vi "Output_RC.vi"(0 "Rack Controller in":refnum<class "Rack Controller.lvclass">, 5 "Output Cluster":T1={"Acknowledgement"={"Actor Enqueuer"=refnum, "VI Reference"=refnum, "VI Name"=""}, "Rack ID"=0, "Clear"=FALSE, "Light Camera Info"={"Light Camera Name"="", " State"=""}, "Camera Optics Diagnostics Result"={"LightCameraName"="", "DiagnosedImage"=refnum, "DustPercentage"=0.0, "Result"=TRUE}, "Receiver Enqueuer"={"Actor Enqueuer"=refnum, "VI Name"=""}, "Error Message"="", "Part Details"={"Part Name"="", "Total Count"=0, "Reel Count"=0}, "Result Cluster"={"RackID"=0, "MeasurementValuesArray "=[], "ImagesArray"=[], "ResultPF"=FALSE, "ProductionCountDetails"={"TotalFail"=0, "TotalPass"=0, "TotalCount"=0}, "ReelCountDetails"={"ReelFail"=0, "ReelPass"=0, "ReelCount"=0}, "ControlPFArray"=[], "SpecificationPFArray"=[], "SpecificationFail"=FALSE, "ReelNumber"=0, "Status"=""}, "Part Info"={"Part Name"="", "Rack ID"=0, "MeasurementIDsArray"=[], "Measurement Names Array"=[], "Spec Values Array"=[], "Camera Names Array"=[], "Total count"=0, "Reel count"=0}, "AllPartInfo"=[{"PartName"="", "NumberOfRacks"=0, "MeasurementIDsArray"=[], "MeasurementNamesArray"=[], "SpecValuesArray"=[]}], "ImagesAndCount"={"Image Array"=[], "ImageCount"=0}}, 7 "Receiver Name":string(combo), 9 "State":string, 11 "error in (no error)":errorcluster) -> (15 "error out":errorcluster)   [LabVIEW 2019, in "Rack Controller.lvclass"]
uses:
  Rack Controller.lvclass
  Inspection Statemachine/Inspection Statemachine Messages/Acknowledgement_SM Msg/Acknowledgement_SM.lvclass
  <vilib>/ActorFramework/Actor/Actor.lvclass
  Inspection Statemachine/Inspection Statemachine Messages/Clear_SM Msg/Clear_SM Msg.lvclass
  Inspection Statemachine/Inspection Statemachine Messages/ErrorMessage_SM Msg/ErrorMessage_SM Msg.lvclass
  Inspection Statemachine/Inspection Statemachine Messages/ResultData_SM Msg/ResultData_SM Msg.lvclass
  <vilib>/ActorFramework/Message Enqueuer/Message Priority.ctl
  <vilib>/ActorFramework/Message Enqueuer/Message Enqueuer.lvclass
  Algorithm/Algorithm Messages/PartInfo_Algo Msg/PartInfo_Algo Msg.lvclass
  Algorithm/Algorithm Messages/StateMessage_Algo Msg/StateMessage_Algo Msg.lvclass
  Algorithm/Algorithm Messages/RackID_Algo Msg/RackID_Algo Msg.lvclass
  Inspection Statemachine/Inspection Statemachine Messages/AllPartInfo_SM Msg/AllPartInfo_SM Msg.lvclass
  Inspection Statemachine/Inspection Statemachine Messages/SensorDiagnosticsResult_SM Msg/SensorDiagnosticsResult_SM Msg.lvclass
  ZenCAM/Camera Controller/Camera Controller Messages/State Message CC Msg/State Message CC Msg.lvclass
  ZenCAM/Camera Controller/Camera Controller Messages/Camera Contoller ID CC Msg/Camera Contoller ID CC Msg.lvclass
  ZenCAM/Camera Controller/Camera Controller Messages/Camera Optics Diagnostics Msg/Camera Optics Diagnostics CC Msg.lvclass
  Inspection Statemachine/Inspection Statemachine Messages/CameraOpticsDiagnosticsResult_SM Msg/CameraOpticsDiagnosticsResult_SM Msg.lvclass
  ZenCAM/Camera Controller/Camera Controller Messages/Reciever Enqueuer CC Msg/Reciever Info CC Msg.lvclass
  ZenCAM/Camera Controller/Camera Controller Messages/Part Name CC Msg/Part Name CC Msg.lvclass
  ZenCAM/Camera Controller/Camera Controller Messages/Run CC Msg/Run CC Msg.lvclass
  Inspection Statemachine/Inspection Statemachine Messages/PartInfoInit_SM Msg/PartInfo_SM Msg.lvclass
  C:/Program Files/National Instruments/LabVIEW 2019/vi.lib/ActorFramework/Actor/Actor.lvclass
  Controls/Output Cluster_RC.ctl
  <vilib>/vision/Image Controls.llb/IMAQ Image.ctl
  Common/Controls/Camera Optics Diagnostics.ctl
  Common/Controls/Camera Optics Diagnostics Result.ctl
  Inspection Statemachine/Controls/Result Cluster_SM.ctl
  Inspection Statemachine/Inspection Statemachine.lvclass
  Common/Controls/AllPartInfo.ctl
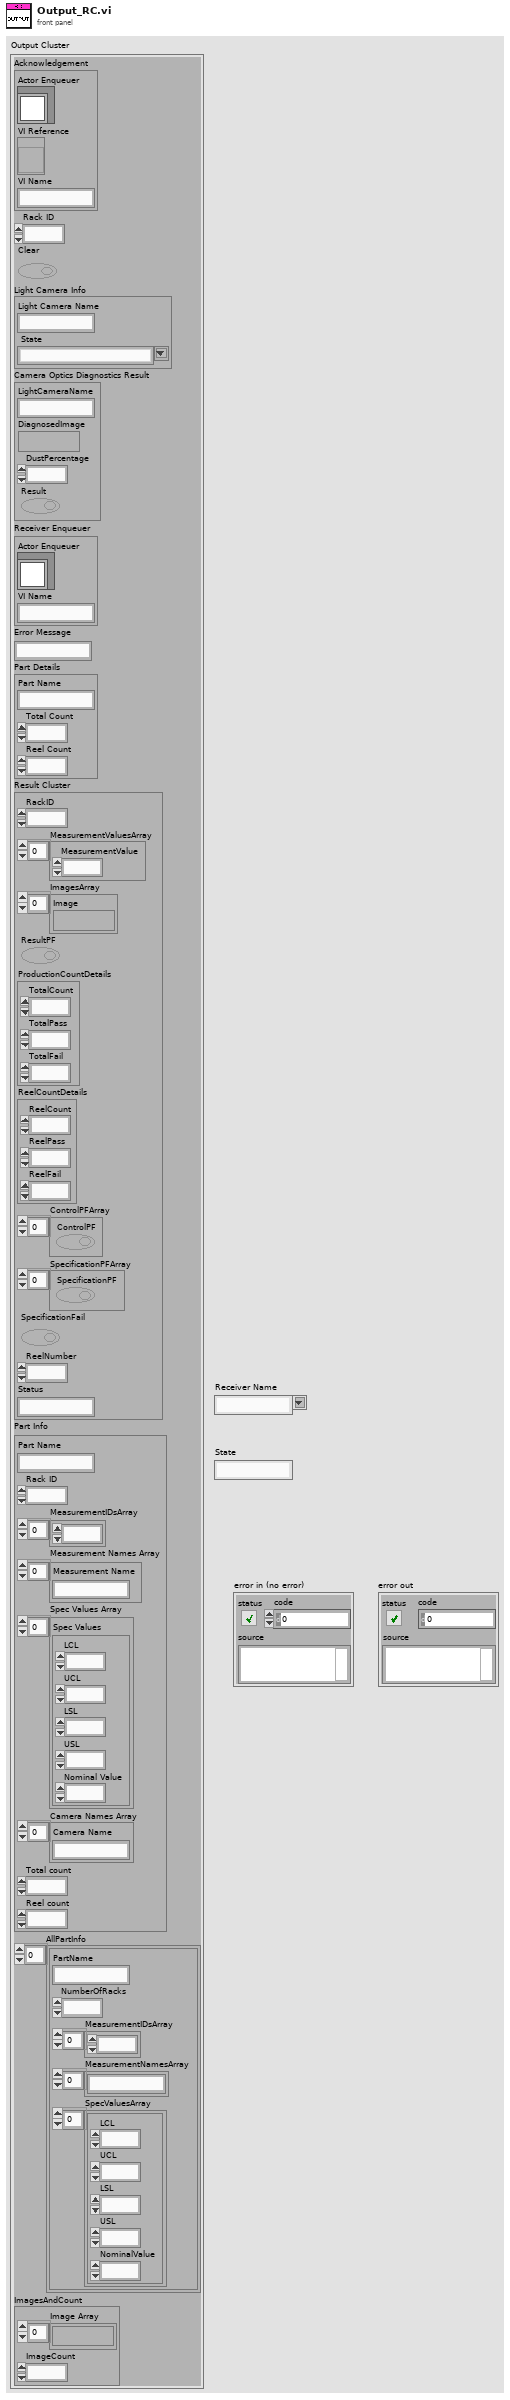
[diagram p1: front panel]
types:
  T1 = typedef "Rack Controller.lvclass/Output Cluster_RC.ctl" = cluster{"Acknowledgement":cluster{"Actor Enqueuer":refnum<class "Message Enqueuer.lvclass">, "VI Reference":refnum<vi>, "VI Name":string}, "Rack ID":u8, "Clear":bool, "Light Camera Info":T2, "Camera Optics Diagnostics Result":T3, "Receiver Enqueuer":cluster{"Actor Enqueuer":refnum<class "Message Enqueuer.lvclass">, "VI Name":string}, "Error Message":string, "Part Details":cluster{"Part Name":string, "Total Count":u64, "Reel Count":u64}, "Result Cluster":T5, "Part Info":cluster{"Part Name":string, "Rack ID":u8, "MeasurementIDsArray":u16[], "Measurement Names Array":string[], "Spec Values Array":cluster{"LCL":dbl, "UCL":dbl, "LSL":dbl, "USL":dbl, "Nominal Value":dbl}[], "Camera Names Array":string[], "Total count":u64, "Reel count":u64}, "AllPartInfo":T6, "ImagesAndCount":cluster{"Image Array":T4[], "ImageCount":u64}}
  T2 = typedef "Camera Optics Diagnostics.ctl" = cluster{"Light Camera Name":string, " State":string}
  T3 = typedef "Camera Optics Diagnostics Result.ctl" = cluster{"LightCameraName":string, "DiagnosedImage":T4, "DustPercentage":dbl, "Result":bool}
  T4 = typedef "IMAQ Image.ctl" = refnum<image>
  T5 = typedef "Inspection Statemachine.lvclass/Result Cluster_SM.ctl" = cluster{"RackID":u8, "MeasurementValuesArray ":dbl[], "ImagesArray":T4[], "ResultPF":bool, "ProductionCountDetails":cluster{"TotalFail":u64, "TotalPass":u64, "TotalCount":u64}, "ReelCountDetails":cluster{"ReelFail":u64, "ReelPass":u64, "ReelCount":u64}, "ControlPFArray":bool[], "SpecificationPFArray":bool[], "SpecificationFail":bool, "ReelNumber":u64, "Status":string}
  T6 = typedef "AllPartInfo.ctl" = cluster{"PartName":string, "NumberOfRacks":u8, "MeasurementIDsArray":u16[], "MeasurementNamesArray":string[], "SpecValuesArray":cluster{"LCL":dbl, "UCL":dbl, "LSL":dbl, "USL":dbl, "NominalValue":dbl}[]}[]
  T7 = typedef "Actor Framework.lvlib/Message Enqueuer.lvclass/Message Priority.ctl" = enum16{"Low", "Normal", "High"}
  T8 = cluster{"State":string, "Image File path":cluster{"Path":path, "Camera ID":i32}[]}
  T9 = cluster{"Reciever Enqueuers":refnum<class "Message Enqueuer.lvclass">, "Recievers Name":string, "Recievers ID":i32}
  T10 = cluster{"Totalcount":u64, "Reelcount":u64, "PartName":string}
  T11 = cluster{"PartName":string, "RackID":u8, "Re-Initialize":bool, "MeasurementIDsArray":u16[], "MeasurementNamesArray":string[], "SpecValuesArray":cluster{"LCL":dbl, "UCL":dbl, "LSL":dbl, "USL":dbl, "NominalValue":dbl}[], "CameraNamesArray":string[]}
  T12 = cluster{"Actor Enqueuer":refnum<class "Message Enqueuer.lvclass">, "VI Reference":refnum<vi>, "VI Name":string}
  T13 = cluster{"LCL":dbl, "UCL":dbl, "LSL":dbl, "USL":dbl, "Nominal Value":dbl}[]
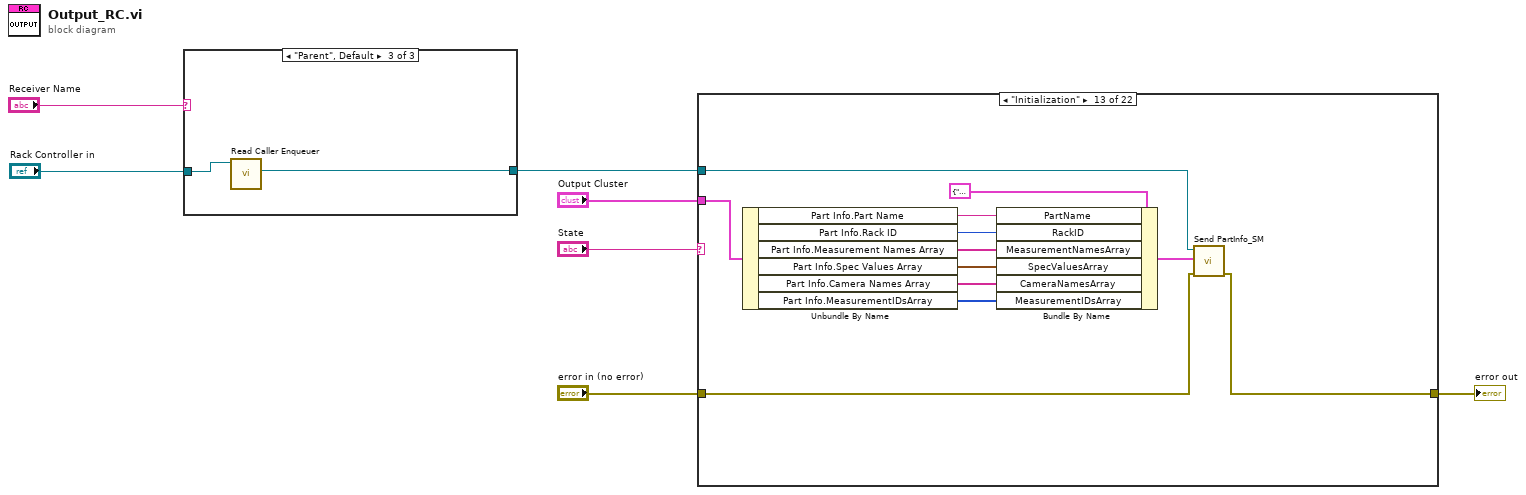
[diagram p0: block diagram]
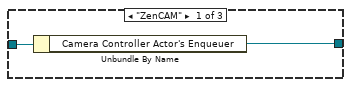
[diagram p2: hidden frame]
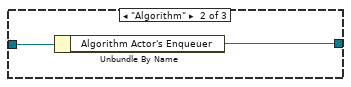
[diagram p3: hidden frame]
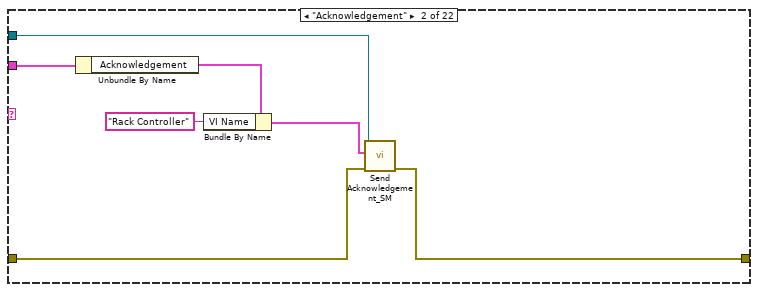
[diagram p5: hidden frame]
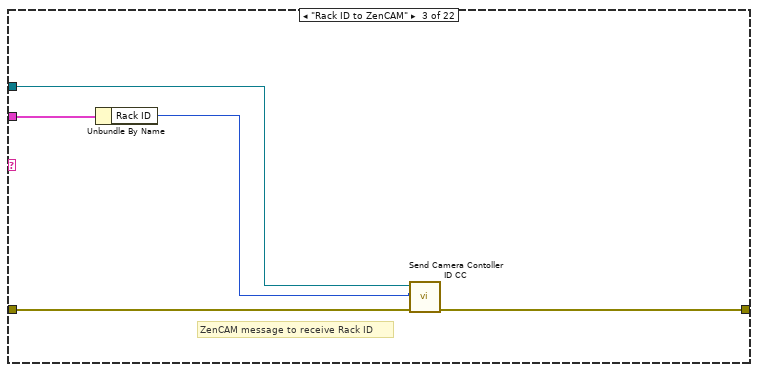
[diagram p6: hidden frame]
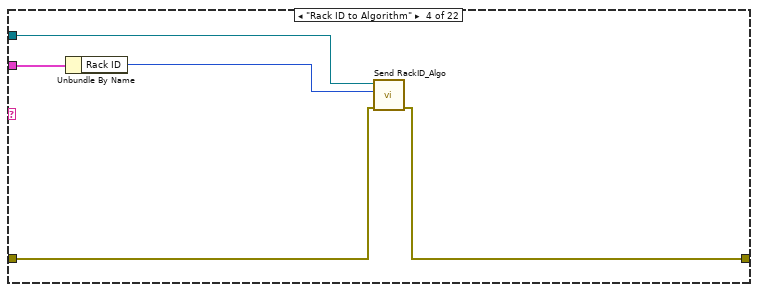
[diagram p7: hidden frame]
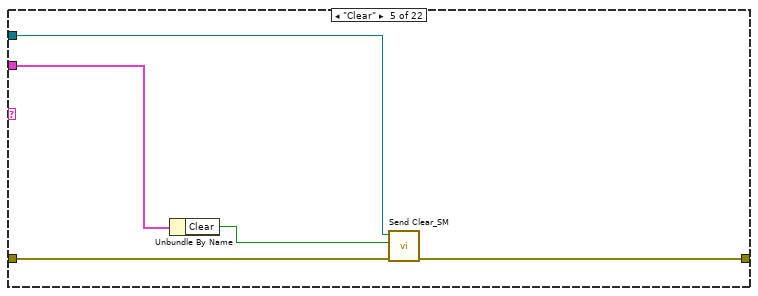
[diagram p8: hidden frame]
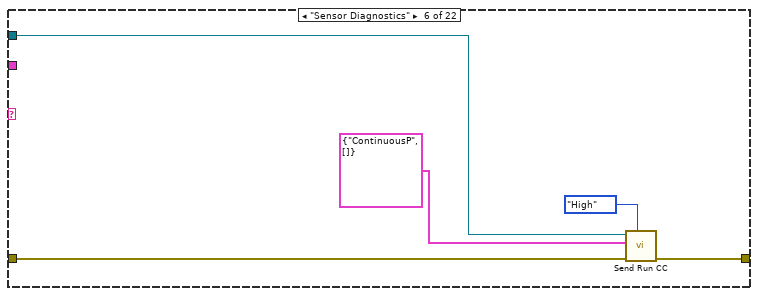
[diagram p9: hidden frame]
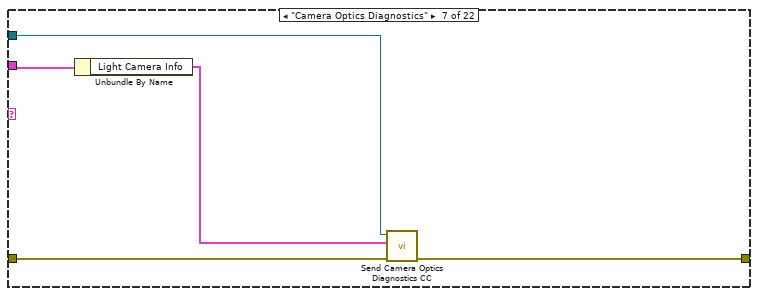
[diagram p10: hidden frame]
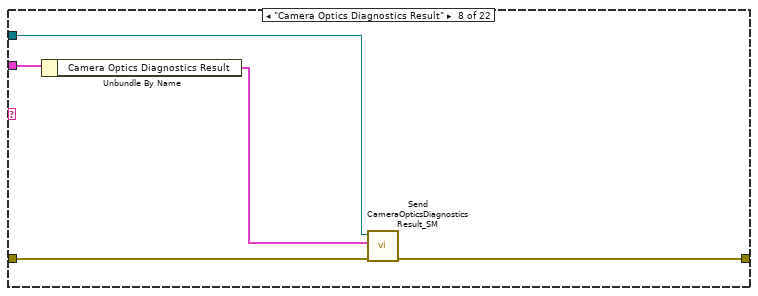
[diagram p11: hidden frame]
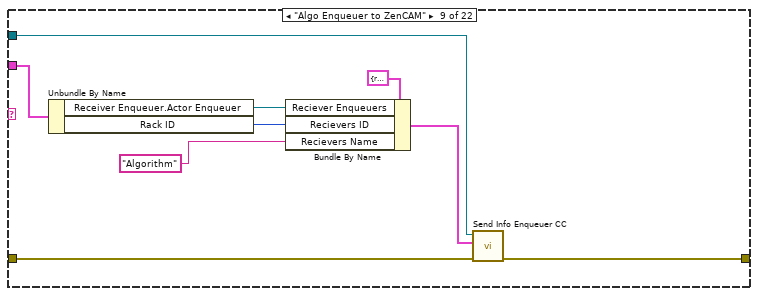
[diagram p12: hidden frame]
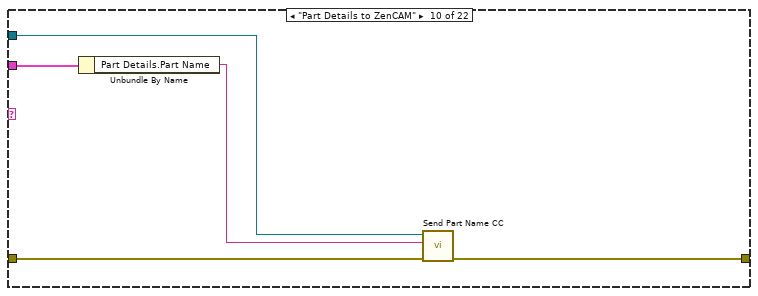
[diagram p13: hidden frame]
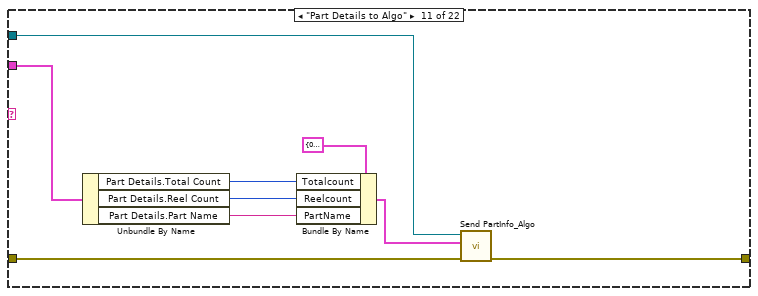
[diagram p14: hidden frame]
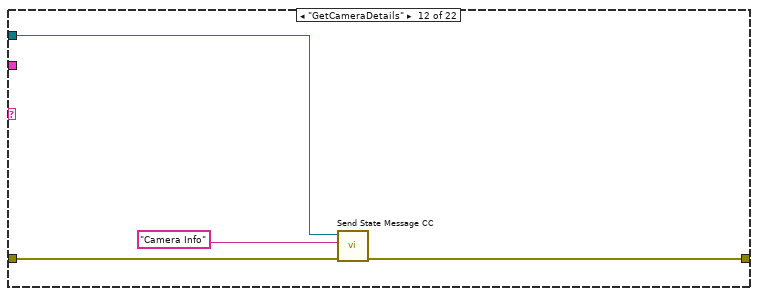
[diagram p15: hidden frame]
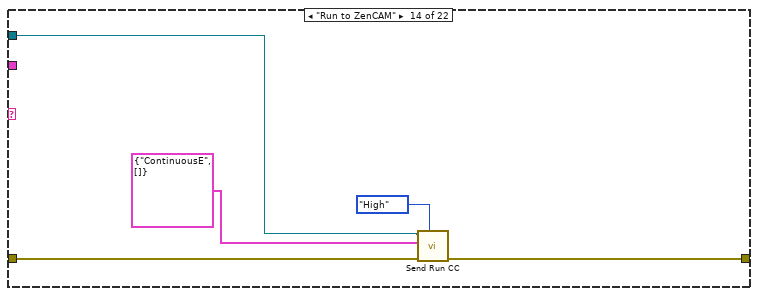
[diagram p16: hidden frame]
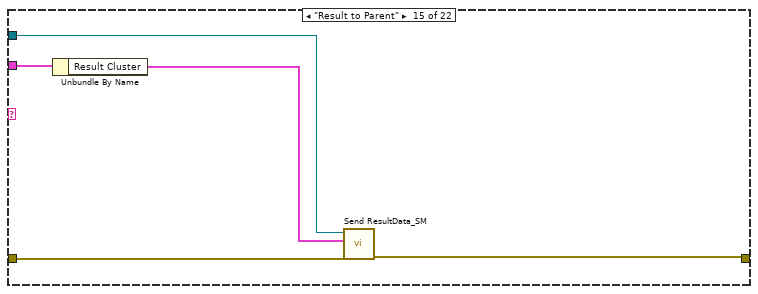
[diagram p17: hidden frame]
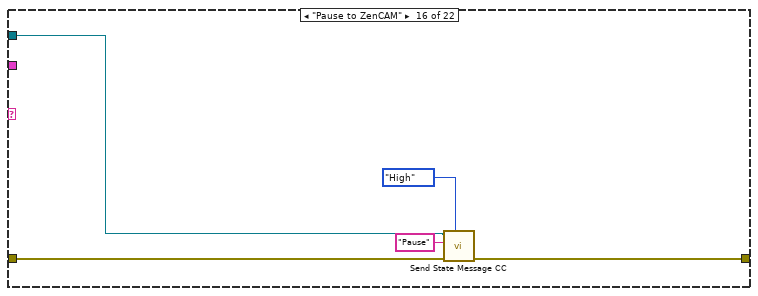
[diagram p18: hidden frame]
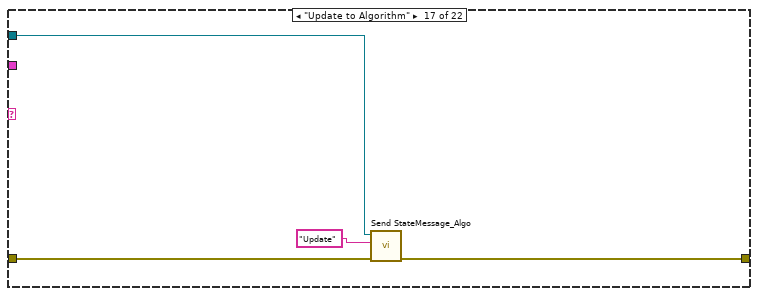
[diagram p19: hidden frame]
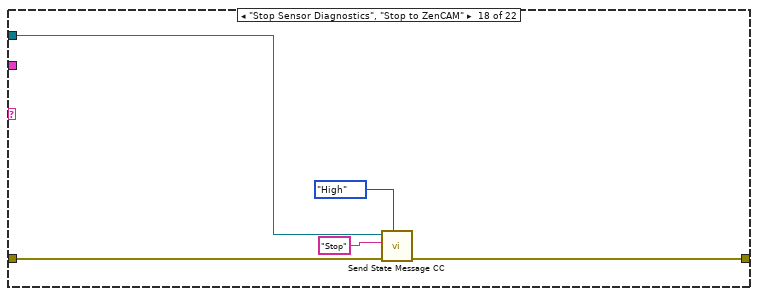
[diagram p20: hidden frame]
diagram:
  n1 = case shown="\"Parent\", Default" "Receiver Name" {
    tunnel: "Rack Controller in" -> [w9 w11 w13]
    tunnel: [w8 w10 w12] -> w4
    frame "ZenCAM" {
      n2 = Unbundle By Name(w9) -> ("Camera Controller Actor's Enqueuer"=w8:refnum<class "Message Enqueuer.lvclass">)
    }
    frame "Algorithm" {
      n3 = Unbundle By Name(w11) -> ("Algorithm Actor's Enqueuer"=w10:refnum<class "Message Enqueuer.lvclass">)
    }
    frame "Parent", Default {
      n4 = call <vilib>:"Read Caller Enqueuer.vi"("Actor"=w13) -> ("Caller Enqueuer"=w12:refnum<class "Message Enqueuer.lvclass">)  [unwired: 10 in]
    }
  }
  n5 = case shown="\"Initialization\"" "State" {
    tunnel: [w14 w21 w24 w27 w35 w39 w44 w49 w54 w63 w71 w77 w88 w94 w99 w104 w108 w113 w118 w122 w125 w130] -> w6
    tunnel: "error in (no error)" -> [w14 w19 w25 w28 w36 w40 w45 w50 w55 w64 w72 w78 w89 w95 w100 w103 w109 w112 w119 w123 w126 w131]
    tunnel: w4 -> [_ w20 w23 w30 w34 w38 w43 w48 w53 w62 w73 w75 w87 w93 w98 w102 w107 w110 w117 w124 w127 w132]
    tunnel: "Output Cluster" -> [_ w18 w26 w31 w33 _ w46 w51 w59 w65 w74 _ w90 _ w97 _ _ _ _ w121 w129 w134]
    frame Default {
    }
    frame "Acknowledgement" {
      n6 = Unbundle By Name(w18) -> ("Acknowledgement"=w17:T12)
      n7 = Bundle By Name(cluster=w17, "VI Name"="Rack Controller") -> (w16:T12)
      n8 = call "Send Acknowledgement_SM.vi"("error in (no error)"=w19, "Acknowledgement"=w16, "Message Enqueuer"=w20) -> ("error out"=w21:errorcluster)  [unwired: 7 in, 1 out]
    }
    frame "Rack ID to ZenCAM" {
      # "ZenCAM message to receive Rack ID"
      n9 = Unbundle By Name(w26) -> ("Rack ID"=w22:u8)
      n10 = call "Send Camera Contoller ID CC.vi"("error in (no error)"=w25, "Camera Controller ID"=w22, "Message Enqueuer"=w23) -> ("error out"=w24:errorcluster)  [unwired: 7 in, 1 out]
    }
    frame "Rack ID to Algorithm" {
      n11 = Unbundle By Name(w31) -> ("Rack ID"=w29:u8)
      n12 = call "Send RackID_Algo.vi"("error in (no error)"=w28, "RackID"=w29, "Message Enqueuer"=w30) -> ("error out"=w27:errorcluster)  [unwired: 7 in, 1 out]
    }
    frame "Clear" {
      n13 = Unbundle By Name(w33) -> ("Clear"=w32:bool)
      n14 = call "Send Clear_SM.vi"("error in (no error)"=w36, "Clear_SM"=w32, "Message Enqueuer"=w34) -> ("error out"=w35:errorcluster)  [unwired: 7 in, 1 out]
    }
    frame "Sensor Diagnostics" {
      n15 = call "Send Run CC.vi"("Message Priority (Normal)"=Message_Priority."High", "error in (no error)"=w40, "Run"=T8 {"State"="ContinuousP", "Image File path"=[]}, "Message Enqueuer"=w38) -> ("error out"=w39:errorcluster)  [unwired: 6 in, 1 out]
    }
    frame "Camera Optics Diagnostics" {
      n16 = Unbundle By Name(w46) -> ("Light Camera Info"=w42:T2)
      n17 = call "Send Camera Optics Diagnostics CC.vi"("error in (no error)"=w45, "Light Camera Info"=w42, "Message Enqueuer"=w43) -> ("error out"=w44:errorcluster)  [unwired: 7 in, 1 out]
    }
    frame "Camera Optics Diagnostics Result" {
      n18 = Unbundle By Name(w51) -> ("Camera Optics Diagnostics Result"=w47:T3)
      n19 = call "Send CameraOpticsDiagnosticsResult_SM.vi"("error in (no error)"=w50, "Camera Optics Diagnostics Result"=w47, "Message Enqueuer"=w48) -> ("error out"=w49:errorcluster)  [unwired: 7 in, 1 out]
    }
    frame "Algo Enqueuer to ZenCAM" {
      n20 = Unbundle By Name(w59) -> ("Receiver Enqueuer.Actor Enqueuer"=w58:refnum<class "Message Enqueuer.lvclass">, "Rack ID"=w56:u8)
      n21 = Bundle By Name(cluster=T9 {"Reciever Enqueuers"=refnum, "Recievers Name"="", "Recievers ID"=0} ("Enqueuer"), "Reciever Enqueuers"=w58, "Recievers ID"=w56, "Recievers Name"="Algorithm" ("Receiver Enqueuer.VI Name")) -> (w52:T9)
      n22 = call "Send Info Enqueuer CC.vi"("error in (no error)"=w55, "Reciever Info"=w52, "Message Enqueuer"=w53) -> ("error out"=w54:errorcluster)  [unwired: 7 in, 1 out]
    }
    frame "Part Details to ZenCAM" {
      n23 = Unbundle By Name(w65) -> ("Part Details.Part Name"=w61:string)
      n24 = call "Send Part Name CC.vi"("error in (no error)"=w64, "Part Name"=w61, "Message Enqueuer"=w62) -> ("error out"=w63:errorcluster)  [unwired: 7 in, 1 out]
    }
    frame "Part Details to Algo" {
      n25 = Unbundle By Name(w74) -> ("Part Details.Total Count"=w70:u64, "Part Details.Reel Count"=w69:u64, "Part Details.Part Name"=w68:string)
      n26 = Bundle By Name(cluster=T10 {"Totalcount"=0, "Reelcount"=0, "PartName"=""} ("PartDetails"), "Totalcount"=w70, "Reelcount"=w69, "PartName"=w68) -> (w66:T10)
      n27 = call "Send PartInfo_Algo.vi"("error in (no error)"=w72, "PartDetails"=w66, "Message Enqueuer"=w73) -> ("error out"=w71:errorcluster)  [unwired: 7 in, 1 out]
    }
    frame "GetCameraDetails" {
      n28 = call "Send State Message CC.vi"("error in (no error)"=w78, "State Message"="Camera Info", "Message Enqueuer"=w75) -> ("error out"=w77:errorcluster)  [unwired: 7 in, 1 out]
    }
    frame "Initialization" {
      n29 = Unbundle By Name(w90) -> ("Part Info.Part Name"=w86:string, "Part Info.Rack ID"=w85:u8, "Part Info.Measurement Names Array"=w84:string[], "Part Info.Spec Values Array"=w83:T13, "Part Info.Camera Names Array"=w82:string[], "Part Info.MeasurementIDsArray"=w79:u16[])
      n30 = Bundle By Name(cluster=T11 {"PartName"="", "RackID"=0, "Re-Initialize"=FALSE, "MeasurementIDsArray"=[], "MeasurementNamesArray"=[], "SpecValuesArray"=[], "CameraNamesArray"=[]} ("PartInfo"), "PartName"=w86, "RackID"=w85, "MeasurementNamesArray"=w84, "SpecValuesArray"=w83, "CameraNamesArray"=w82, "MeasurementIDsArray"=w79) -> (w80:T11)
      n31 = call "Send PartInfo_SM.vi"("error in (no error)"=w89, "PartInfo"=w80, "Message Enqueuer"=w87) -> ("error out"=w88:errorcluster)  [unwired: 7 in, 1 out]
    }
    frame "Run to ZenCAM" {
      n32 = call "Send Run CC.vi"("Message Priority (Normal)"=Message_Priority."High", "error in (no error)"=w95, "Run"=T8 {"State"="ContinuousE", "Image File path"=[]}, "Message Enqueuer"=w93) -> ("error out"=w94:errorcluster)  [unwired: 6 in, 1 out]
    }
    frame "Result to Parent" {
      n33 = Unbundle By Name(w97) -> ("Result Cluster"=w96:T5)
      n34 = call "Send ResultData_SM.vi"("error in (no error)"=w100, "Result Cluster"=w96, "Message Enqueuer"=w98) -> ("error out"=w99:errorcluster)  [unwired: 7 in, 1 out]
    }
    frame "Pause to ZenCAM" {
      n35 = call "Send State Message CC.vi"("Message Priority (Normal)"=Message_Priority."High", "error in (no error)"=w103, "State Message"="Pause", "Message Enqueuer"=w102) -> ("error out"=w104:errorcluster)  [unwired: 6 in, 1 out]
    }
    frame "Update to Algorithm" {
      n36 = call "Send StateMessage_Algo.vi"("error in (no error)"=w109, "StateMessage"="Update", "Message Enqueuer"=w107) -> ("error out"=w108:errorcluster)  [unwired: 7 in, 1 out]
    }
    frame "Stop Sensor Diagnostics", "Stop to ZenCAM" {
      n37 = call "Send State Message CC.vi"("Message Priority (Normal)"=Message_Priority."High", "error in (no error)"=w112, "State Message"="Stop", "Message Enqueuer"=w110) -> ("error out"=w113:errorcluster)  [unwired: 6 in, 1 out]
    }
    frame "Stop to Algorithm" {
      n38 = call "Send StateMessage_Algo.vi"("Message Priority (Normal)"=Message_Priority."High", "error in (no error)"=w119, "StateMessage"="Stop", "Message Enqueuer"=w117) -> ("error out"=w118:errorcluster)  [unwired: 6 in, 1 out]
    }
    frame "Error Message" {
      n39 = Unbundle By Name(w121) -> ("Error Message"=w120:string)
      n40 = call "Send ErrorMessage_SM.vi"("error in (no error)"=w123, "Error Message"=w120, "Message Enqueuer"=w124) -> ("error out"=w122:errorcluster)  [unwired: 7 in, 1 out]
    }
    frame "AllPartInfo" {
      n41 = Unbundle By Name(w129) -> ("AllPartInfo"=w128:T6)
      n42 = call "Send AllPartInfo_SM.vi"("error in (no error)"=w126, "AllPartInfo"=w128, "Message Enqueuer"=w127) -> ("error out"=w125:errorcluster)  [unwired: 7 in, 1 out]
    }
    frame "SensorDiagnosticsResult" {
      n43 = Unbundle By Name(w134) -> ("ImagesAndCount"=w133:cluster{"Image Array":T4[], "ImageCount":u64})
      n44 = call "Send SensorDiagnosticsResult_SM.vi"("error in (no error)"=w131, "ImagesAndCount"=w133, "Message Enqueuer"=w132) -> ("error out"=w130:errorcluster)  [unwired: 7 in, 1 out]
    }
  }
  "error out" <- w6
